vi "XML Report_Init.vi"(8 "error in (no error)":errorcluster) -> (0 "error out":errorcluster, 3 "XML_Report out":refnum<class "XML Report.lvclass">)   [LabVIEW 2011, in "XML Report.lvclass"]
doc: "This VI defines the object type for a XML Report.\n\nAAL 9/09"
uses:
  XML Report.lvclass
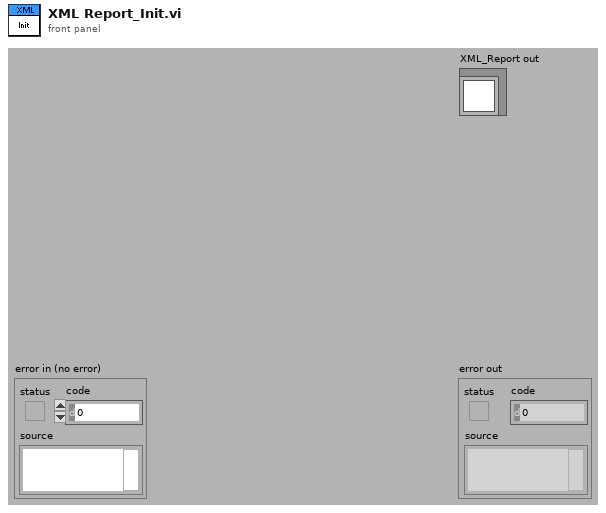
[diagram p1: front panel]
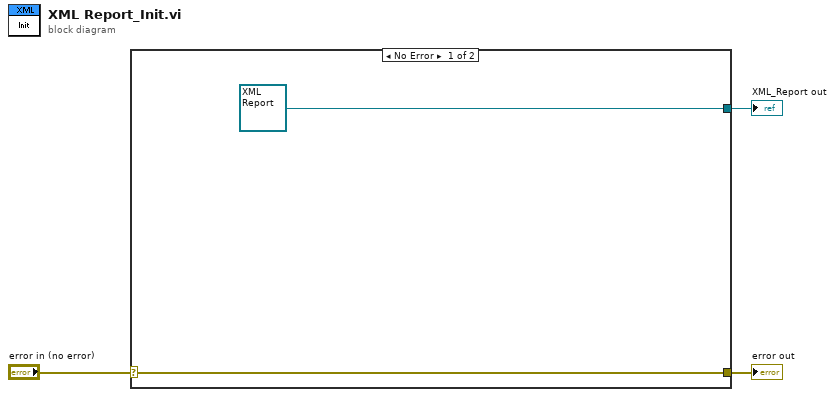
[diagram p0: block diagram]
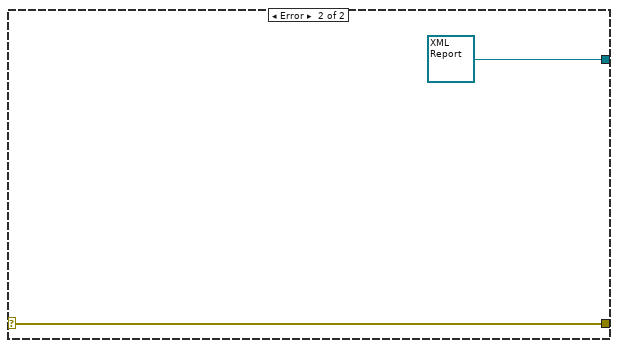
[diagram p2: hidden frame]
diagram:
  n1 = case shown="No Error" "error in (no error)" {
    selector: "error in (no error)" -> [w4 w7]
    tunnel: [w4 w7] -> w2
    tunnel: [refnum<class "XML Report.lvclass"> refnum ("TXT_Report.lvclass") refnum<class "XML Report.lvclass"> refnum ("TXT_Report.lvclass")] -> w1
    frame No Error {
    }
    frame Error {
    }
  }
  "error out" <- w2
  "XML_Report out" <- w1
